vi "Read Variant (sta).vi"(11 "Test Object in":refnum<class "Test Object.lvclass">) -> (2 "Variant":variant, 3 "Test Object out":refnum<class "Test Object.lvclass">)   [LabVIEW 2015, in "Test Object.lvclass"]
uses:
  Test Object.lvclass
  Test Object.lvclass/Test Object.ctl
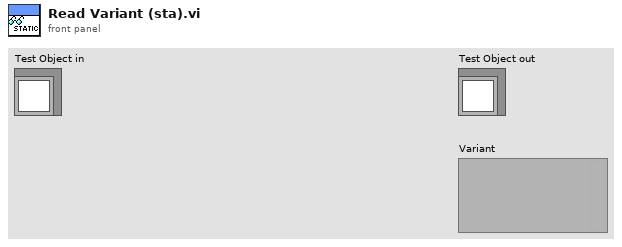
[diagram p1: front panel]
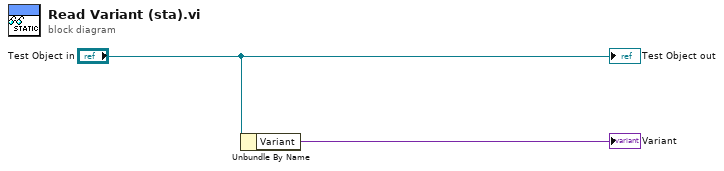
[diagram p0: block diagram]
diagram:
  n1 = Unbundle By Name("Test Object in") -> ("Variant"=→"Variant":variant)
  "Test Object out" <- "Test Object in"
